vi "Shutdown.vi"(8 "error in (no error)":errorcluster, 11 "H-Intfc in":refnum<class "REST Interface.lvclass">) -> (0 "error out":errorcluster, 3 "H-Intfc out":refnum<class "REST Interface.lvclass">)   [LabVIEW 2018, in "REST Interface.lvlib" / "REST Interface.lvclass"]
uses:
  REST Interface.lvclass
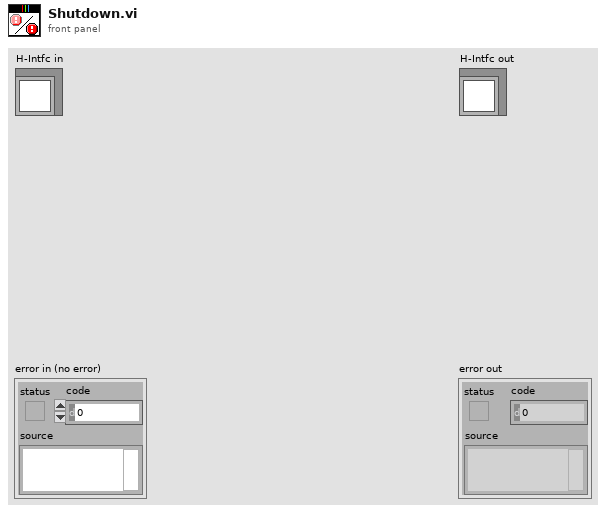
[diagram p1: front panel]
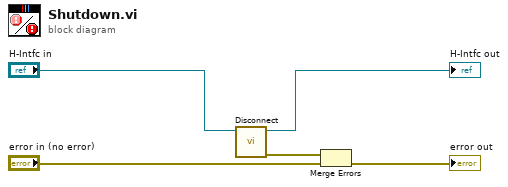
[diagram p0: block diagram]
diagram:
  n1 = call-dynamic "Disconnect.vi"("H-Intfc in"="H-Intfc in") -> ("error out"=w1:errorcluster, "H-Intfc out"=→"H-Intfc out":refnum<class "REST Interface.lvclass">)  [unwired: 9 in]
  n2 = Merge Errors(w1, "error in (no error)") -> (→"error out":errorcluster)
